vi "Read Stamp Slot.vi"(8 "error in (no error)":errorcluster, 10 "Stamp Slot":i32, 11 "WorkTable Class in":refnum<class "WorkTable Class.lvclass">) -> (0 "error out":errorcluster, 2 "Stamp Slot":T1, 3 "WorkTable Class out":refnum<class "WorkTable Class.lvclass">)   [LabVIEW 2011, in "WorkTable Class.lvclass"]
uses:
  WorkTable Class.lvclass
  Type Definitions/Worktable_Stamp.ctl
  Vec3d Class/Vec3d Class.lvclass
  Orient3d Class/Orient3d Class.lvclass
  Utils/Type Definitions/Position_Orientation.ctl
  Config Manager Class/Type Definitions/Stamp Type.ctl
  WorkTable Class.lvclass/WorkTable Class.ctl
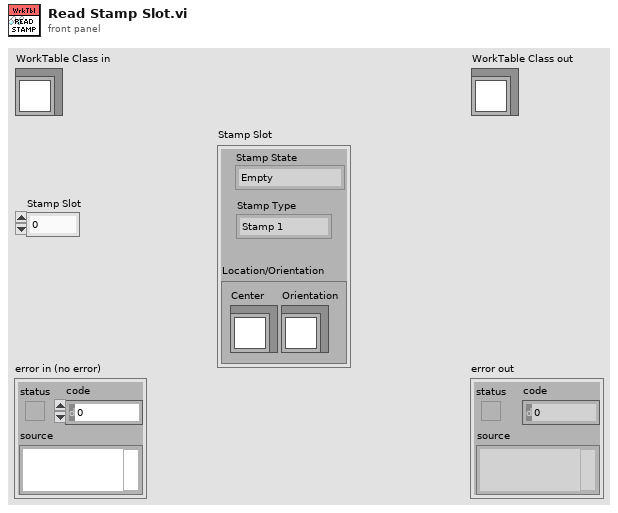
[diagram p1: front panel]
types:
  T1 = typedef "Worktable_Stamp.ctl" = cluster{"Stamp State":enum16{"Empty", "Populated", "Used"}, "Location/Orientation":T2, "Stamp Type":T3}
  T2 = typedef "Position_Orientation.ctl" = cluster{"Center":refnum<class "Vec3d Class.lvclass">, "Orientation":refnum<class "Orient3d Class.lvclass">}
  T3 = typedef "Stamp Type.ctl" = enum16{"Stamp 1", "Stamp 2", "Stamp 3", "Stamp 4", "Stamp 5"}
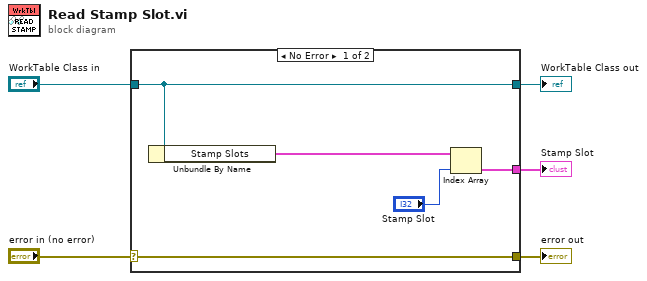
[diagram p0: block diagram]
diagram:
  n1 = case shown="No Error" "error in (no error)" {
    selector: "error in (no error)" -> [w10 w11]
    tunnel: [w10 w11] -> w4
    tunnel: [w9 w12] -> w2
    tunnel: "WorkTable Class in" -> [w9 w12]
    tunnel: [w6 _] -> w1
    frame No Error {
      n2 = Unbundle By Name(w9) -> ("Stamp Slots"=w8:T1[])
      n3 = Index Array(array=w8, index="Stamp Slot") -> (element=w6:T1)
    }
    frame Error {
    }
  }
  "error out" <- w4
  "WorkTable Class out" <- w2
  "Stamp Slot" <- w1
